vi "WIDTH_DIV_4.vi"() -> (0 "WIDTH_DIV_4":i16=100)   [LabVIEW 2020]
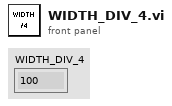
[diagram p1: front panel]
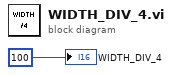
[diagram p0: block diagram]
diagram:
  "WIDTH_DIV_4" <- i16 100
